vi "SetRemarks_popup.vi"(2 "Input Line Command":string, 3 "error in (no error)":errorcluster) -> (8 "Cancel":bool, 9 "Output Line Command":string, 10 "error out":errorcluster)   [LabVIEW 2020]
panel:
  in  "platform":u16(ring) items=["Mac", "PC"]
  in  "Cancel Button":bool
  in  "OK Button":bool
  in  "Remarks":string
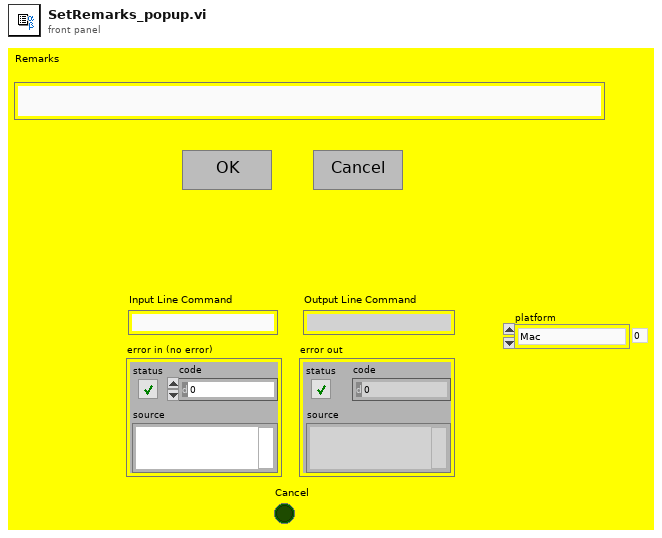
[diagram p1: front panel]
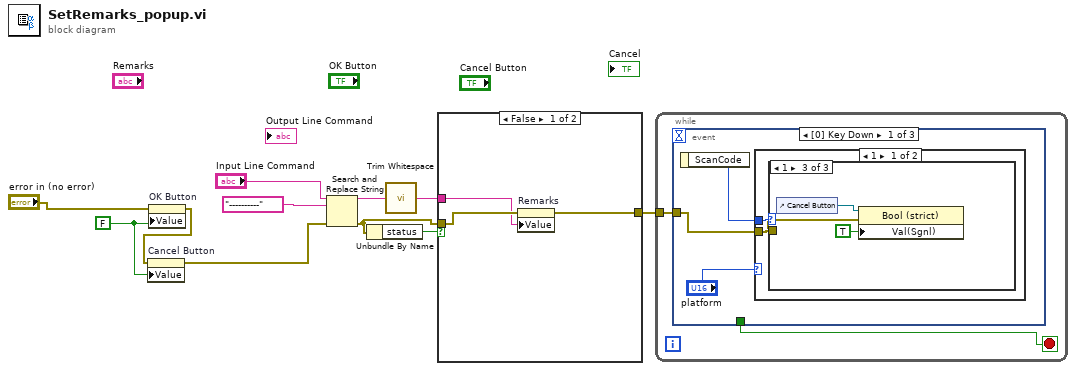
[diagram p0: block diagram]
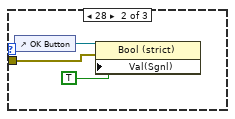
[diagram p3: hidden frame]
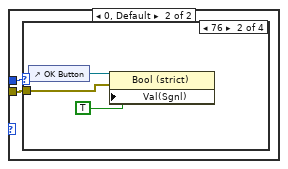
[diagram p4: hidden frame]
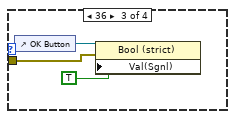
[diagram p6: hidden frame]
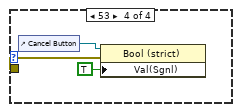
[diagram p7: hidden frame]
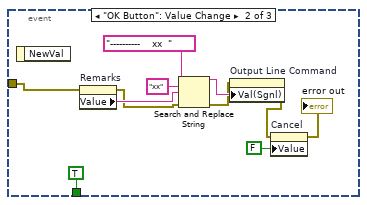
[diagram p8: hidden frame]
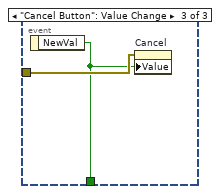
[diagram p9: hidden frame]
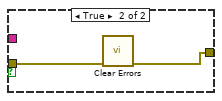
[diagram p10: hidden frame]
diagram:
  w11 = FALSE
  n1 = property on="OK Button" class="Bool (strict)"(error in="error in (no error)", "Value"=w11) -> (error out=w9:errorcluster)  [unwired: 1 in, 1 out]
  n2 = property on="Cancel Button" class="Bool (strict)"(error in=w9, "Value"=w11) -> (error out=w8:errorcluster)  [unwired: 1 in, 1 out]
  n3 = Search and Replace String(input string="Input Line Command", search string="----------", error in=w8) -> (result string=w5:string, error out=w3:errorcluster)  [unwired: 5 in, 2 out]
  n4 = Unbundle By Name(w3) -> ("status"=w4:bool)
  n5 = call <vilib>:"Trim Whitespace.vi"("string"=w5) -> ("trimmed string"=w2:string)  [unwired: 1 in]
  n6 = case shown="False" w4 {
    tunnel: w3 -> [w14 w16]
    tunnel: w2 -> [w13 _]
    tunnel: [w12 w15] -> w1
    frame False {
      n7 = property on="Remarks" class="Str"(error in=w14, "Value"=w13) -> (error out=w12:errorcluster)  [unwired: 1 in, 1 out]
    }
    frame True {
      n8 = call <vilib>:"Clear Errors.vi"("error in (no error)"=w16) -> ("error out"=w15:errorcluster)  [unwired: 5 in, 1 out]
    }
  }
  n9 = while {
    tunnel: w1 -> [w18]
    stop <- w17 stop-if-true
    n10 = event shown="[0] Key Down" {
      selector: _ -> [_ _ _]
      dyn-events: _ -> [_ _ _]
      timeout: _ -> [_ _ _]
      tunnel: w18 -> [w20 w48 w53]
      tunnel: [_ TRUE ("NewVal") w52] -> w17
      event Key Down {
        n11 = event-data() -> ("ScanCode"=w21:i16)  [unwired: 1 in]
        n12 = case shown="1" "platform" {
          tunnel: w21 -> [w23 w31]
          tunnel: w20 -> [w22 w30]
          frame 1 {
            n13 = case shown="1" w23 {
              tunnel: w22 -> [_ w25 w28]
              frame Default {
              }
              frame 28 {
                n14 = control-ref of="OK Button"() -> (w26:refnum<vi>)
                n15 = property on="Property Node" class="Bool (strict)"(reference=w26, error in=w25, "Val(Sgnl)"=TRUE ("Value (Signaling)")) -> ()  [unwired: 2 out]
              }
              frame 1 {
                n16 = control-ref of="Cancel Button"() -> (w29:refnum<vi>)
                n17 = property on="Property Node" class="Bool (strict)"(reference=w29, error in=w28, "Val(Sgnl)"=TRUE ("Value (Signaling)")) -> ()  [unwired: 2 out]
              }
            }
          }
          frame 0, Default {
            n18 = case shown="76" w31 {
              tunnel: w30 -> [_ w33 w36 w39]
              frame Default {
              }
              frame 76 {
                n19 = control-ref of="OK Button"() -> (w34:refnum<vi>)
                n20 = property on="Property Node" class="Bool (strict)"(reference=w34, error in=w33, "Val(Sgnl)"=TRUE ("Value (Signaling)")) -> ()  [unwired: 2 out]
              }
              frame 36 {
                n21 = control-ref of="OK Button"() -> (w37:refnum<vi>)
                n22 = property on="Property Node" class="Bool (strict)"(reference=w37, error in=w36, "Val(Sgnl)"=TRUE ("Value (Signaling)")) -> ()  [unwired: 2 out]
              }
              frame 53 {
                n23 = control-ref of="Cancel Button"() -> (w40:refnum<vi>)
                n24 = property on="Property Node" class="Bool (strict)"(reference=w40, error in=w39, "Val(Sgnl)"=TRUE ("Value (Signaling)")) -> ()  [unwired: 2 out]
              }
            }
          }
        }
      }
      event "OK Button": Value Change {
        n25 = event-data() -> ()  [unwired: 1 in, 1 out]
        n26 = property on="Remarks" class="Str"(error in=w48) -> (error out=w47:errorcluster, "Value"=w49:string)  [unwired: 1 in, 1 out]
        n27 = Search and Replace String(input string="----------    xx  ", search string="xx", replace string=w49, error in=w47) -> (result string=w46:string, error out=w45:errorcluster)  [unwired: 4 in, 2 out]
        n28 = property on="Output Line Command" class="Str"(error in=w45, "Val(Sgnl)"=w46) -> (error out=w42:errorcluster)  [unwired: 1 in, 1 out]
        n29 = property on="Cancel" class="Bool (strict)"(error in=w42, "Value"=FALSE ("Cancel")) -> (error out=→"error out":errorcluster)  [unwired: 1 in, 1 out]
      }
      event "Cancel Button": Value Change {
        n30 = event-data() -> ("NewVal"=w52:bool)  [unwired: 1 in]
        n31 = property on="Cancel" class="Bool (strict)"(error in=w53, "Value"=w52) -> ()  [unwired: 1 in, 2 out]
      }
    }
  }
